vi "opencvSegmentVisualize.vi"(1 "XY":u16[][][](array[numeric]), 2 "ImgIn":u16[][][](array[numeric])) -> ()   [LabVIEW 2017]
uses:
  globalUtilities.vi
panel:
  out "Intensity Graph":u16[][](graph)
  in  "dotsize":i32=3
  in  "index (page)":i32
  in  "stop":bool
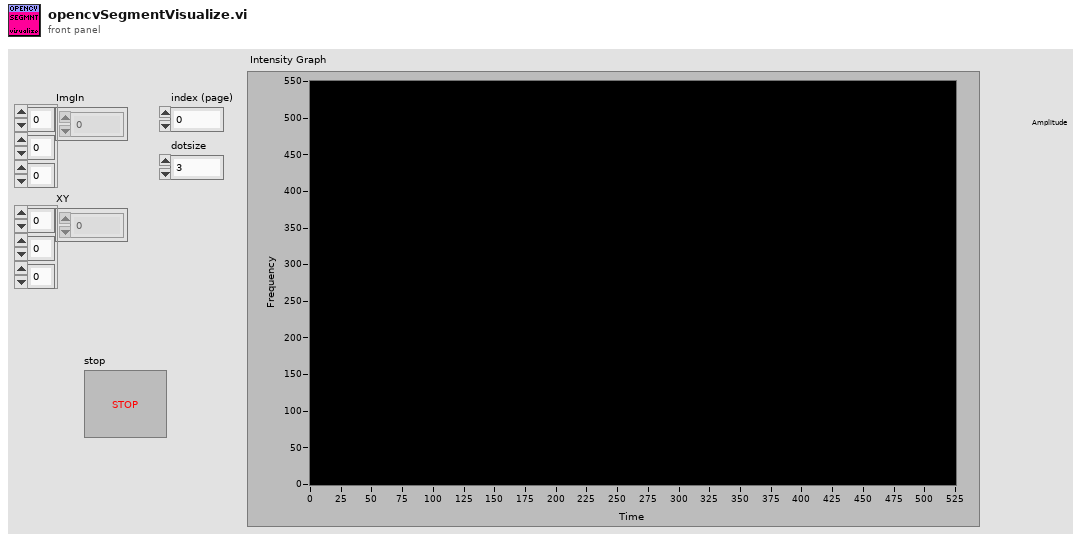
[diagram p1: front panel]
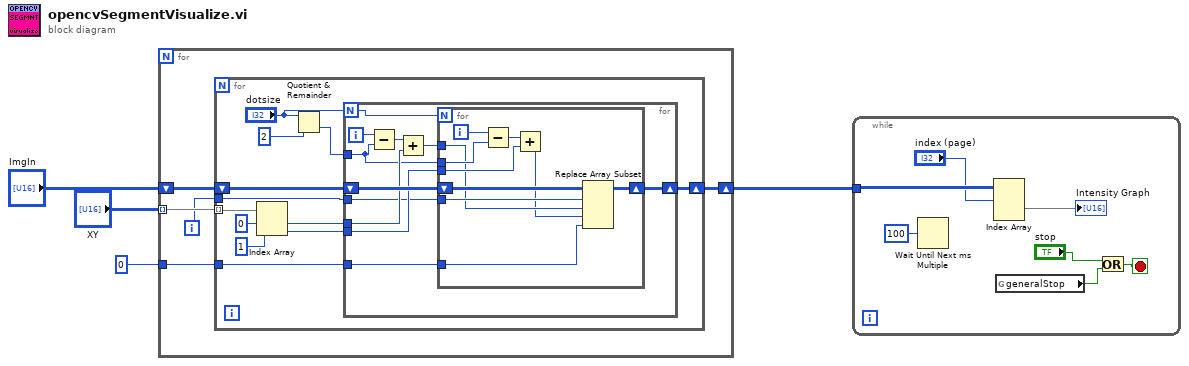
[diagram p0: block diagram]
diagram:
  n1 = for {
    shift-right: [w6] -> w4
    shift-left: "ImgIn" -> [w8]
    tunnel: "XY" -> [w9] mode=indexing
    tunnel: u16 0 ("new element/subarray") -> [w5]
    i -> [w7]
    n2 = for {
      tunnel: w9 -> [w21] mode=indexing
      shift-right: [w10] -> w6
      shift-left: w8 -> [w13]
      tunnel: w7 -> [w12]
      tunnel: w5 -> [w11]
      n3 = Index Array(array=w21, index #1=0 ("index"), index #2=1 ("index")) -> (element #1=w17:u16, element #2=w16:u16)
      n4 = Quotient & Remainder(x="dotsize", y=2) -> (floor(x/y)=w14:i32)  [unwired: 1 out]
      n5 = for {
        N: "dotsize" -> [w32]
        tunnel: w17 -> [w28]
        tunnel: w16 -> [w26]
        tunnel: w14 -> [w27]
        shift-right: [w22] -> w10
        shift-left: w13 -> [w30]
        tunnel: w12 -> [w25]
        tunnel: w11 -> [w23]
        i -> [w31]
        n6 = Subtract(x=w31, y=w27) -> (x-y=w29:i32)
        n7 = Add(x=w29, y=w28) -> (x+y=w24:i32)
        n8 = for {
          N: w32 -> [_]
          shift-right: [w37] -> w22
          shift-left: w30 -> [w38]
          tunnel: w27 -> [w41]
          tunnel: w26 -> [w39]
          tunnel: w25 -> [w36]
          tunnel: w24 -> [w35]
          tunnel: w23 -> [w33]
          i -> [w42]
          n9 = Subtract(x=w42, y=w41) -> (x-y=w40:i32)
          n10 = Add(x=w40, y=w39) -> (x+y=w34:i32)
          n11 = Replace Array Subset(array=w38, new element=w33, index (dim 0)=w36, index (dim 1)=w35, index (dim 2)=w34) -> (w37:u16[][][])
        }
      }
    }
  }
  n12 = while {
    tunnel: w4 -> [w49]
    stop <- w43 stop-if-true
    n13 = Wait Until Next ms Multiple(millisecond multiple=u32 100) -> ()  [unwired: 1 out]
    n14 = Index Array(array=w49, index (dim 0)="index (page)") -> (element=→"Intensity Graph":u16[][])  [unwired: 2 in]
    n15 = global read "globalUtilities.vi" "generalStop"() -> (w45:bool)
    n16 = Or(x="stop", y=w45) -> (x .or. y?=w43:bool)
  }
